vi "GlobalLaserOnOff.vi"() -> ()   [LabVIEW 2011]
panel:
  in  "OnOffLaser":bool
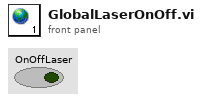
[diagram p1: front panel]
diagram:
